vi "_RT_FPGA_Main.vi"(6 "Timeout":i32, 7 "Function":T1, 8 "Error in":errorcluster, 9 "U64EventCodes":u64[](array[numeric]), 10 "U64ScanData_in":u64[](array[numeric]), 11 "Data_in":variant) -> (0 "Error out":errorcluster, 1 "SigData_out":i16[](array[numeric]), 3 "Data out":variant)   [LabVIEW 2018]
uses:
  PublicSubVI/Ctl/_ctl_RT_FPGA_Function.ctl
  <vilib>/FPGAPlugInAG/sbRIO-9627/niLvFpga_Close_sbRIO-9627.vi
  <vilib>/FPGAPlugInAG/sbRIO-9627/niLvFpga_Open_sbRIO-9627.vi
  <vilib>/FPGAPlugInAG/sbRIO-9627/niLvFpga_Reset_sbRIO-9627.vi
  <vilib>/FPGAPlugInAG/sbRIO-9627/niLvFpga_Run_sbRIO-9627.vi
  <vilib>/Utility/error.llb/Error Cluster From Error Code.vi
  <vilib>/rvi/errors/niLvFpgaAdjustHostInterfaceError.vi
  <vilib>/rvi/interface/common/niFpgaWaitOnOcc.vi
  <vilib>/rvi/interface/nirviCloseFPGA/nirviCloseFPGA.xnode
  FPGA Bitfiles/ATIQITAnalyser_FPGAZynq7020_FPGAMainv7.lvbitx
  <vilib>/rvi/interface/nirviOpenFPGA/nirviOpenFPGA.xnode
  <vilib>/rvi/interface/nirviMethod/nirviMethod.xnode
  <vilib>/rvi/interface/nirviReadWriteControl/nirviReadWriteControl.xnode
  <vilib>/rvi/errors/niLvFpgaMergeErrorWithErrorCode.vi
  FPGA Bitfiles/ATIQITAnalyser_FPGATarget_FPGAMainv6.lvbitx
  FPGA/FPGA_Main_v6.vi
  NiFpgaLv.dll
  <vilib>/FPGAPlugInAG/sbRIO-9627/niLvFpga_StopFifo_sbRIO-9627.vi
  <vilib>/FPGAPlugInAG/sbRIO-9627/niLvFpga_ConfigureFifo_sbRIO-9627.vi
  <vilib>/FPGAPlugInAG/sbRIO-9627/niLvFpga_WriteFifo_sbRIO-9627.vi
  <vilib>/FPGAPlugInAG/sbRIO-9627/niLvFpga_StartFifo_sbRIO-9627.vi
  <vilib>/FPGAPlugInAG/sbRIO-9627/niLvFpga_ReadFifo_sbRIO-9627.vi
panel:
  out "EventCode":u8=255
  out "EventCode Ele#":u32
  out "RFU64 Ele#":u32
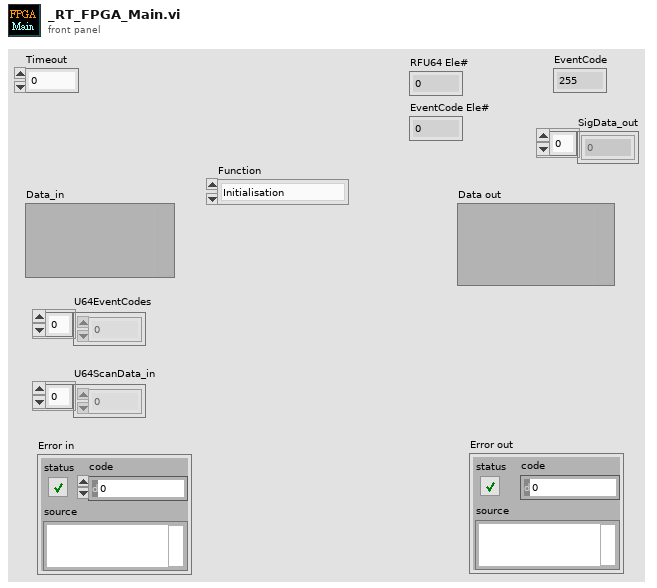
[diagram p1: front panel]
types:
  T1 = typedef "_ctl_RT_FPGA_Function.ctl" = enum16{"Initialisation", "Execution", "Digital In"}
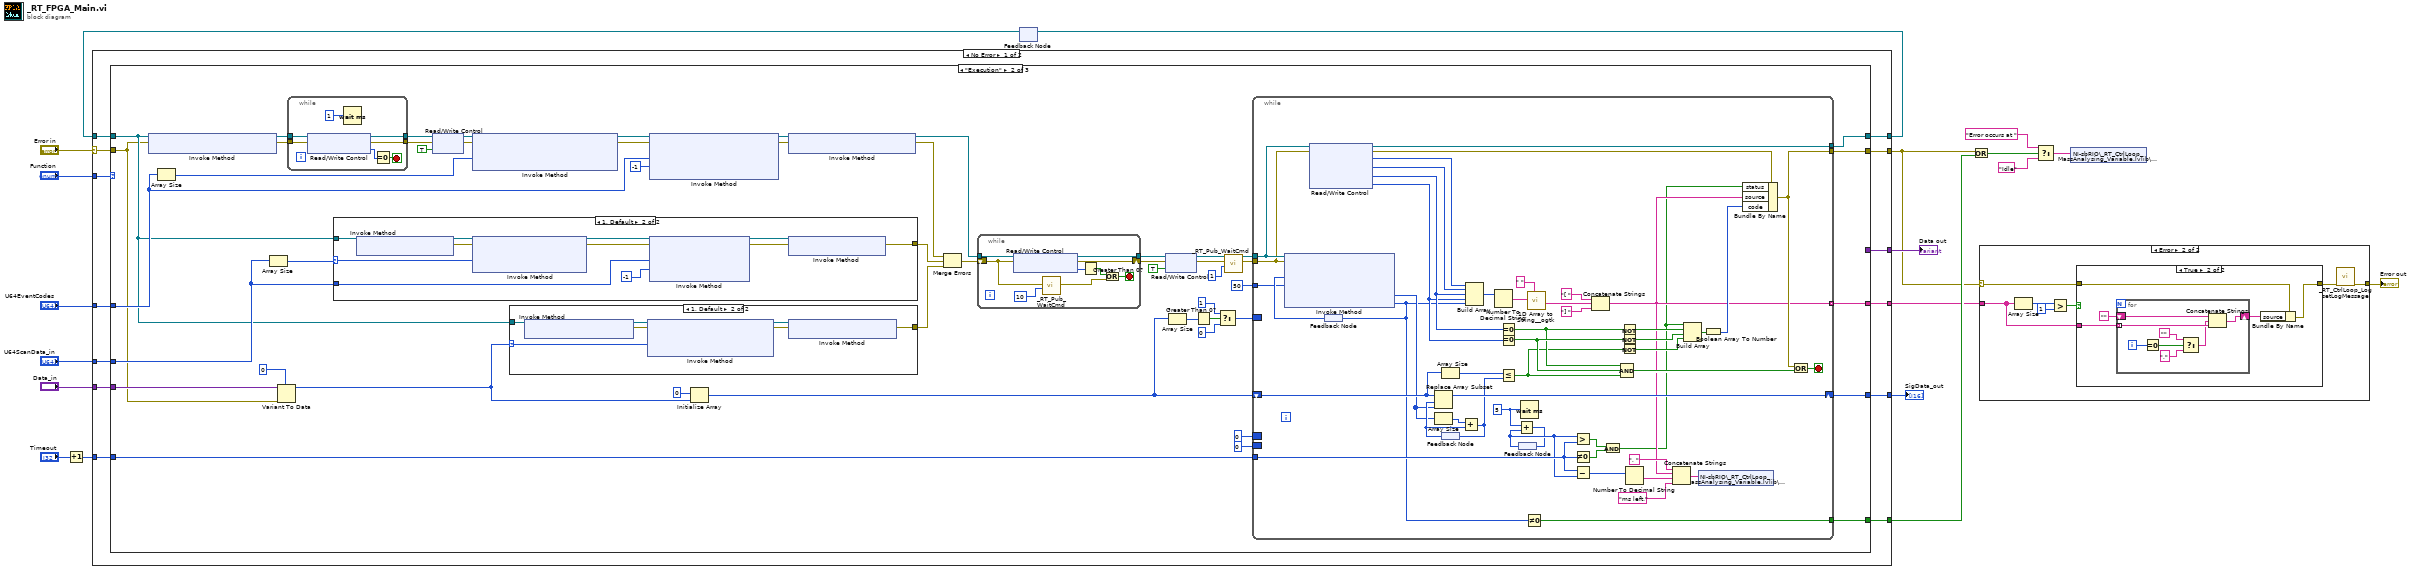
[diagram p0: block diagram]
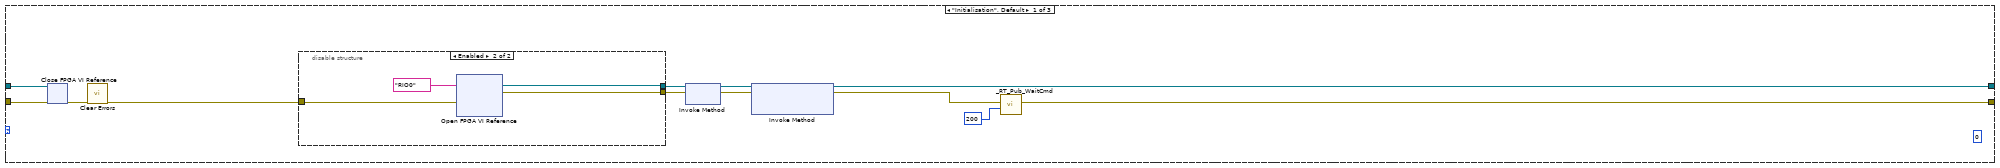
[diagram p4: hidden frame]
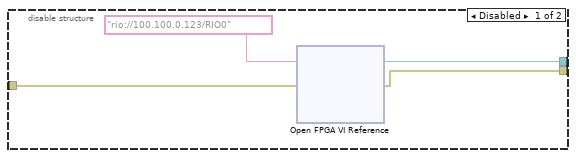
[diagram p5: hidden frame]
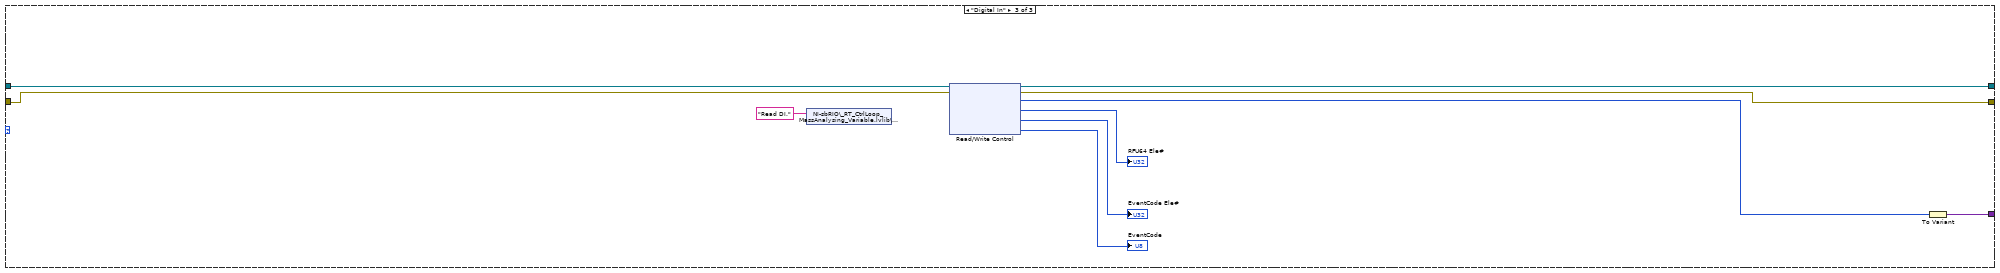
[diagram p8: hidden frame]
diagram:
  n1 = Increment(x="Timeout") -> (x+1=w8:i32)
  n2 = feedback #1() -> (w17:refnum<k20>)  [unwired: 1 in]
  n3 = case shown="No Error" "Error in" {
    selector: "Error in" -> [w28 w195]
    tunnel: "Function" -> [w32 _]
    tunnel: [w21 w196] -> w18
    tunnel: w17 -> [w31 w196]
    tunnel: [w20 w195] -> w2
    tunnel: "Data_in" -> [w30 _]
    tunnel: "U64ScanData_in" -> [w29 _]
    tunnel: "U64EventCodes" -> [w27 _]
    tunnel: [w26 _] -> w12
    tunnel: [w25 _] -> w11
    tunnel: w8 -> [w24 _]
    tunnel: [w23 _] -> w6
    tunnel: [w22 _] -> w3
    frame No Error {
      n4 = case shown="\"Execution\"" w32 {
        tunnel: [w33 w88 w193] -> w21
        tunnel: w31 -> [w44 w71 w194]
        tunnel: [w34 w55 w186] -> w20
        tunnel: w28 -> [w43 w63 w185]
        tunnel: w30 -> [_ w100 _]
        tunnel: w29 -> [_ w95 _]
        tunnel: w27 -> [_ w98 _]
        tunnel: [_ w86 _] -> w26
        tunnel: [_ _ w191] -> w25
        tunnel: w24 -> [_ w73 _]
        tunnel: [_ w68 _] -> w23
        tunnel: [_ w54 _] -> w22
        frame "Initialisation", Default {
          (unwired) u16 0 ("N2")
          n5 = xnode "Close FPGA VI Reference"("FPGA VI Reference In"=w44, "error in"=w43) -> ("error out"=w42:errorcluster)
          n6 = call <vilib>:"Clear Errors.vi"("error in (no error)"=w42) -> ("error out"=w41:errorcluster)  [unwired: 5 in, 1 out]
          n7 = disable-structure shown="Enabled" {
            disable-tunnel: w41 -> [w47 w50]
            disable-tunnel: [w46 w52] -> w40
            disable-tunnel: [w45 w51] -> w39
            frame Disabled {
              n8 = xnode "Open FPGA VI Reference"("error in"=w47, "resource name"=tag "rio://100.100.0.123/RIO0") -> ("FPGA VI Reference Out"=w46:refnum<k20>, "error out"=w45:errorcluster)
            }
            frame Enabled {
              n9 = xnode "Open FPGA VI Reference"("error in"=w50, "resource name"=tag "RIO0") -> ("FPGA VI Reference Out"=w52:refnum<k20>, "error out"=w51:errorcluster)
            }
          }
          n10 = xnode "Invoke Method"("FPGA VI Reference In"=w40, "error in"=w39) -> ("FPGA VI Reference Out"=w38:refnum<k20>, "error out"=w37:errorcluster)
          n11 = xnode "Invoke Method"("FPGA VI Reference In"=w38, "error in"=w37) -> ("FPGA VI Reference Out"=w33:refnum<k20>, "error out"=w35:errorcluster)  [unwired: 1 in]
          n12 = call "_RT_Pub_WaitCmd.vi"("milliseconds to wait"=u32 200, "error in (no error)"=w35) -> ("error out"=w34:errorcluster)  [unwired: 9 in]
        }
        frame "Execution" {
          n13 = xnode "Invoke Method"("FPGA VI Reference In"=w71, "error in"=w63) -> ("FPGA VI Reference Out"=w64:refnum<k20>, "error out"=w67:errorcluster)
          n14 = Array Size(array=w98) -> (size(s)=w101:i32)
          n15 = Array Size(array=w95) -> (size(s)=w76:i32)
          n16 = Variant To Data(error in=w63, type=0, Variant=w100) -> (data=w75:i32)  [unwired: 1 out]
          n17 = while {
            tunnel: w64 -> [w105]
            tunnel: [w106] -> w65
            tunnel: w67 -> [w108]
            tunnel: [w107] -> w66
            stop <- w104 stop-if-true
            n18 = xnode "Read/Write Control"("FPGA VI Reference In"=w105, "error in"=w108) -> ("FPGA VI Reference Out"=w106:refnum<k20>, "error out"=w107:errorcluster, "EventCode Ele#"=w103:u32)
            n19 = Wait (ms)(milliseconds to wait=u32 1) -> ()  [unwired: 1 out]
            n20 = Equal To 0?(x=w103) -> (x = 0?=w104:bool)
          }
          n21 = case shown="1, Default" w76 {
            selector: w76 -> [_ w116]
            tunnel: w95 -> [_ w124]
            tunnel: [_ w120] -> w91
            tunnel: w71 -> [_ w117]
            frame 0 {
            }
            frame 1, Default {
              n22 = xnode "Invoke Method"("FPGA VI Reference In"=w117) -> ("FPGA VI Reference Out"=w119:refnum<k20>, "error out"=w118:errorcluster)  [unwired: 1 in]
              n23 = xnode "Invoke Method"("FPGA VI Reference In"=w119, "error in"=w118, "Requested Depth"=w116) -> ("FPGA VI Reference Out"=w126:refnum<k20>, "error out"=w125:errorcluster)  [unwired: 1 out]
              n24 = xnode "Invoke Method"("FPGA VI Reference In"=w126, "error in"=w125, "Data"=w124, "Timeout (ms)"=-1) -> ("FPGA VI Reference Out"=w123:refnum<k20>, "error out"=w122:errorcluster)  [unwired: 1 out]
              n25 = xnode "Invoke Method"("FPGA VI Reference In"=w123, "error in"=w122) -> ("error out"=w120:errorcluster)  [unwired: 1 out]
            }
          }
          n26 = xnode "Read/Write Control"("FPGA VI Reference In"=w65, "error in"=w66, "Reset"=TRUE) -> ("FPGA VI Reference Out"=w70:refnum<k20>, "error out"=w69:errorcluster)
          n27 = xnode "Invoke Method"("FPGA VI Reference In"=w70, "error in"=w69, "Requested Depth"=w101) -> ("FPGA VI Reference Out"=w97:refnum<k20>, "error out"=w96:errorcluster)  [unwired: 1 out]
          n28 = case shown="1, Default" w75 {
            selector: w75 -> [_ w112]
            tunnel: [_ w113] -> w90
            tunnel: w71 -> [_ w109]
            frame 0 {
            }
            frame 1, Default {
              n29 = xnode "Invoke Method"("FPGA VI Reference In"=w109) -> ("FPGA VI Reference Out"=w110:refnum<k20>, "error out"=w111:errorcluster)  [unwired: 1 in]
              n30 = xnode "Invoke Method"("FPGA VI Reference In"=w110, "error in"=w111, "Requested Depth"=w112) -> ("FPGA VI Reference Out"=w115:refnum<k20>, "error out"=w114:errorcluster)  [unwired: 1 out]
              n31 = xnode "Invoke Method"("FPGA VI Reference In"=w115, "error in"=w114) -> ("error out"=w113:errorcluster)  [unwired: 1 out]
            }
          }
          n32 = xnode "Invoke Method"("FPGA VI Reference In"=w97, "error in"=w96, "Data"=w98, "Timeout (ms)"=-1) -> ("FPGA VI Reference Out"=w94:refnum<k20>, "error out"=w93:errorcluster)  [unwired: 1 out]
          n33 = Initialize Array(i16 0, w75) -> (w80:i16[])
          n34 = xnode "Invoke Method"("FPGA VI Reference In"=w94, "error in"=w93) -> ("FPGA VI Reference Out"=w53:refnum<k20>, "error out"=w89:errorcluster)
          n35 = Merge Errors(w89, w91, w90) -> (w61:errorcluster)
          n36 = while {
            shift-right: [w128] -> w83
            shift-left: w61 -> [w127]
            tunnel: w53 -> [w134]
            tunnel: [w131] -> w78
            stop <- w130 stop-if-true
            n37 = xnode "Read/Write Control"("FPGA VI Reference In"=w134, "error in"=w127) -> ("FPGA VI Reference Out"=w131:refnum<k20>, "error out"=w128:errorcluster, "EventCode Ele#"=w133:u32)
            n38 = call "_RT_Pub_WaitCmd.vi"("milliseconds to wait"=u32 10, "error in (no error)"=w127) -> ("error out"=w129:errorcluster)  [unwired: 9 in]
            n39 = Greater Than 0?(x=w133) -> (x > 0?=w132:bool)
            n40 = Or(x=w132, y=w129) -> (x .or. y?=w130:bool)
          }
          n41 = xnode "Read/Write Control"("FPGA VI Reference In"=w78, "error in"=w83, "Start"=TRUE) -> ("FPGA VI Reference Out"=w85:refnum<k20>, "error out"=w60:errorcluster)
          n42 = Array Size(array=w80) -> (size(s)=w79:i32)
          n43 = Greater Than 0?(x=w79) -> (x > 0?=w57:bool)
          n44 = Select(t=u32 1, s=w57, f=u32 0) -> (s? t:f=w56:u32)
          n45 = call "_RT_Pub_WaitCmd.vi"("milliseconds to wait"=u32 1, "error in (no error)"=w60) -> ("error out"=w81:errorcluster)  [unwired: 9 in]
          n46 = while {
            shift-right: [w184] -> w86
            shift-left: w80 -> [w180]
            tunnel: w85 -> [w139]
            tunnel: [w137] -> w88
            tunnel: [w160] -> w55
            border: 0 -> [_]
            border: w56 -> [_]
            tunnel: w81 -> [w138]
            border: u32 0 ("y") -> [_]
            tunnel: w73 -> [w158]
            tunnel: [w170] -> w68
            tunnel: 50 ("Timeout (ms)") -> [w169]
            tunnel: [w141] -> w54 mode=indexing
            stop <- w179 stop-if-true
            w157 = u32 5 ("milliseconds to wait")
            n47 = xnode "Read/Write Control"("FPGA VI Reference In"=w139, "error in"=w138) -> ("FPGA VI Reference Out"=w137:refnum<k20>, "error out"=w136:errorcluster, "EventCode"=w152:u8, "SubEventCode"=w151:u8, "EventCode Ele#"=w150:u32, "RFU64 Ele#"=w149:u32)
            n48 = feedback #2() -> (w183:u32)
            n49 = xnode "Invoke Method"("FPGA VI Reference In"=w139, "error in"=w138, "Number of Elements"=w183, "Timeout (ms)"=w169) -> ("Data"=w178:i16[], "Elements Remaining"=w148:u32)  [unwired: 2 out]
            n50 = feedback-in #2(w148) -> ()
            n51 = Array Size(array=w178) -> (size(s)=w182:i32)
            n52 = feedback #3() -> (w181:i32)
            n53 = Replace Array Subset(array=w180, new element=w178, index=w181) -> (w184:i16[])
            n54 = Array Size(array=w180) -> (size(s)=w154:i32)
            n55 = Add(x=w182, y=w181) -> (x+y=w153:i32)
            n56 = feedback-in #3(w153) -> ()
            n57 = Build Array(w152, w151, w150, w149, w148) -> (w142:u32[])
            n58 = Number To Decimal String(number=w142) -> (decimal integer string=w147:string[])  [unwired: 1 in]
            n59 = Equal To 0?(x=w150) -> (x = 0?=w167:bool)
            n60 = Equal To 0?(x=w149) -> (x = 0?=w168:bool)
            n61 = Less Or Equal?(x=w154, y=w153) -> (x <= y?=w166:bool)
            n62 = feedback #4() -> (w156:u32)
            n63 = Add(x=w157, y=w156) -> (x+y=w155:u32)
            n64 = feedback-in #4(w155) -> ()
            n65 = Wait (ms)(milliseconds to wait=w157) -> ()  [unwired: 1 out]
            n66 = Not Equal To 0?(x=w148) -> (x != 0?=w170:bool)
            n67 = call <userlib>:"1D Array to String__ogtk.vi"("delimiter (Tab)"=" ", "Array of Strings"=w147) -> ("delimited string"=w143:string)  [unwired: 9 in]
            n68 = Greater?(x=w156, y=w158) -> (0:w176:bool)
            n69 = Not Equal To 0?(x=w158) -> (x != 0?=w175:bool)
            n70 = Subtract(x=w158, y=w156) -> (x-y=w172:u32)
            n71 = Concatenate Strings("[ " ("FirmwareStatus"), w143, "] " ("string")) -> (w141:string)
            n72 = And(x=w176, y=w175) -> (x .and. y?=w140:bool)
            n73 = Not(x=w167) -> (.not. x?=w165:bool)
            n74 = Not(x=w168) -> (.not. x?=w164:bool)
            n75 = Not(x=w166) -> (.not. x?=w163:bool)
            n76 = Compound Arithmetic op=AND(w167, w168, w166) -> (w177:bool)
            n77 = Number To Decimal String(number=w172) -> (decimal integer string=w171:string)  [unwired: 1 in]
            n78 = Concatenate Strings(", " ("FirmwareStatus"), w141, w171, "ms left." ("string")) -> (w174:string)
            n79 = Build Array(w140, w165, w164, w163) -> (w162:bool[])
            n80 = shared-variable "NI-sbRIO\\_RT_CtrlLoop_MassAnalysing_Variable.lvlib\\FirmwareStatus"(w174) -> ()  [unwired: 1 in, 1 out]
            n81 = Boolean Array To Number(Boolean array=w162) -> (number=w161:u32)
            n82 = Bundle By Name(cluster=w136, "status"=w140, "source"=w141, "code"=w161) -> (w160:errorcluster)
            n83 = Compound Arithmetic op=OR(w160, w177) -> (w179:bool)
          }
        }
        frame "Digital In" {
          n84 = shared-variable "NI-sbRIO\\_RT_CtrlLoop_MassAnalysing_Variable.lvlib\\FirmwareStatus"("Read DI." ("FirmwareStatus")) -> ()  [unwired: 1 in, 1 out]
          n85 = xnode "Read/Write Control"("FPGA VI Reference In"=w194, "error in"=w185) -> ("FPGA VI Reference Out"=w193:refnum<k20>, "error out"=w186:errorcluster, "DI"=w192:u8, "RFU64 Ele#"=→"RFU64 Ele#":u32, "EventCode Ele#"=→"EventCode Ele#":u32, "EventCode"=→"EventCode":u8)
          n86 = To Variant(anything=w192) -> (Variant=w191:variant)
        }
      }
    }
    frame Error {
    }
  }
  "SigData_out" <- w12
  "Data out" <- w11
  n87 = feedback-in #1(w18) -> ()
  n88 = Or(x=w2, y=w6) -> (x .or. y?=w7:bool)
  n89 = case shown="Error" w2 {
    selector: w2 -> [w197 w200]
    tunnel: w3 -> [_ w204]
    tunnel: [w197 w198] -> w1
    frame No Error {
    }
    frame Error {
      n90 = Array Size(array=w204) -> (size(s)=w203:i32)
      n91 = Greater?(x=w203, y=1) -> (0:w201:bool)
      n92 = case shown="True" w201 {
        tunnel: w204 -> [_ w208]
        tunnel: w200 -> [w205 w207]
        tunnel: [w205 w206] -> w199
        frame False {
        }
        frame True {
          n93 = for {
            tunnel: w208 -> [w218] mode=indexing
            shift-right: [w211] -> w209
            shift-left: "" -> [w217]
            i -> [w216]
            n94 = Equal To 0?(x=w216) -> (x = 0?=w215:bool)
            n95 = Select(t="", s=w215, f=",") -> (s? t:f=w212:string)
            n96 = Concatenate Strings(w217, w212, w218) -> (w211:string)
          }
          n97 = Bundle By Name(cluster=w207, "source"=w209) -> (w206:errorcluster)
        }
      }
      n98 = call "_RT_CtrlLoop_Log setLogMessage.vi"("error in"=w199) -> ("error out"=w198:errorcluster)  [unwired: 9 in, 1 out]
    }
  }
  "Error out" <- w1
  n99 = Select(t="Error occurs at ", s=w7, f="Idle") -> (s? t:f=w10:string)
  n100 = shared-variable "NI-sbRIO\\_RT_CtrlLoop_MassAnalysing_Variable.lvlib\\FirmwareStatus"(w10) -> ()  [unwired: 1 in, 1 out]
